vi "Acoustic Frequency Response Chirp.vi"(0 "TSM context":T1, 1 "dB SPL":dbl=94.0 format="%#_13g", 2 "Response Frequency (Hz)":dbl[](array[numeric])=[300.0, 18000.0], 5 "Start Freq (Hz)":dbl=20.0 format="%#_13g", 7 "Stop Freq (Hz)":dbl=20000.0 format="%#_13g", 9 "Samples":i32=128) -> (15 "error out":errorcluster)   [LabVIEW 2020]
doc: "VI performs an Acoustic Frequency Test with Calibrated Chirp waveform as input stimulus to microphone to obtain the equivalent Voltage Amplitude at given Frequencies."
uses:
  <vilib>/NI_TestStand_SemiconductorModule/NI_TestStand_Semiconductor_Module.lvlibp/PinMap/General/SemiconductorModuleContext.ctl
  e949006d-0b04-4f52-9731-e8b82caba12d.vi
  4e50633a-216a-4e31-9721-602c2020261f.vi
  c74fba9a-7462-4997-8ba2-8448d8120d66.vi
  f7f5d33f-d09a-4d82-ae73-b91c36f905d8.vi
  85eadde2-c8f2-4106-bb4c-7373345d24d2.vi
  28004d85-2d46-4c01-a9b5-50f3a10d13bf.vi
  e949006d-0b04-4f52-9731-e8b82caba12d.vi/1878dca8-edba-410e-aa20-92364f789876.vi
  4e50633a-216a-4e31-9721-602c2020261f.vi/75bb260e-55ca-447c-884a-a6f6cf63e709.vi
  <vilib>/measure/matone.llb/Extract Single Tone Information N Chan.vi
  <vilib>/NI_TestStand_SemiconductorModule/NI_TestStand_Semiconductor_Module.lvlibp/PinMap/General/Publish/PublishDataDoubleFunctionalTest.vi
  <vilib>/NI_TestStand_SemiconductorModule/NI_TestStand_Semiconductor_Module.lvlibp
  <vilib>/measure/NI_MAPro.lvlib
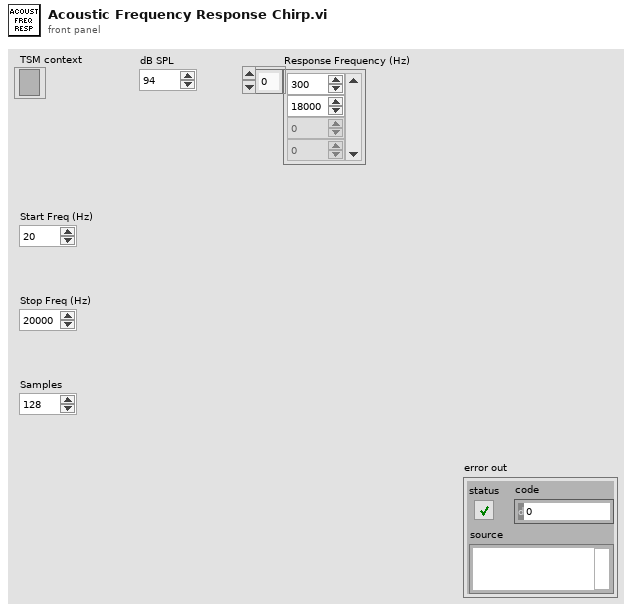
[diagram p1: front panel]
types:
  T1 = typedef "NI_TestStand_Semiconductor_Module.lvlibp/SemiconductorModuleContext.ctl" = refnum<k7>
  T2 = typedef "TSM DAQmx Multi-Task.ctl" = cluster{"Pin Query Context":refnum<class "MultiplePinMultipleSessionQueryContext.lvclass">, "SSC":T3[], "Site Numbers":i32[], "Pins":tag[]}
  T3 = typedef "SSC DAQmx.ctl" = cluster{"DAQmx Task ":refnum<k21>, "Channels":string, "Channel Lists":string}
  T4 = cluster{"approx freq. (optional)":dbl, "search (+/- % of Fsampl.)":dbl}
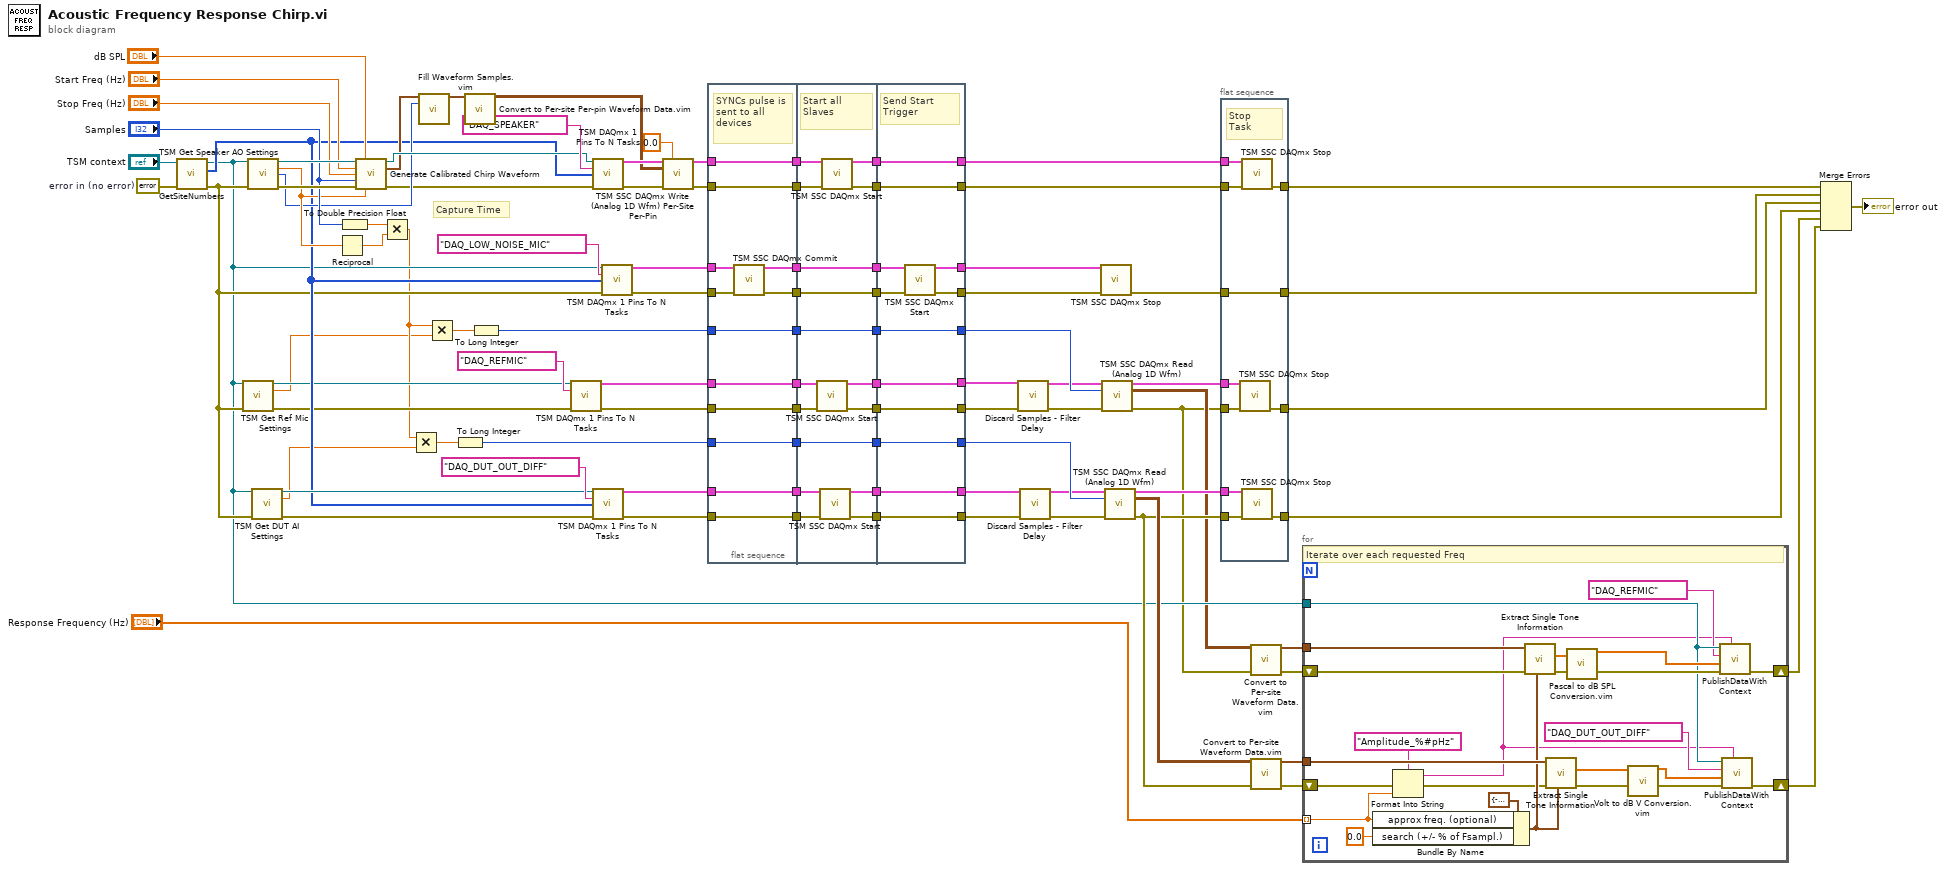
[diagram p0: block diagram]
diagram:
  w73 = errorcluster {"status"=FALSE, "code"=0, "source"=""}  # error in (no error)
  # "Capture Time"
  n1 = call <vilib>:"GetSiteNumbers.vi"("error in (no error)"=w73, "Semiconductor Module Context"="TSM context") -> ("error out"=w33:errorcluster, "Site Numbers"=w36:i32[], "Semiconductor Module Context Out"=w32:T1)  [unwired: 6 in, 1 out]
  n2 = call "TSM Get Ref Mic Settings.vi"("TSM context"=w32, "error in (no error)"=w33) -> ("TSM context Out"=w28:T1, "Sampling Rate (Hz)"=w25:dbl, "error out"=w30:errorcluster)  [unwired: 8 in, 3 out]
  n3 = call "TSM Get Speaker AO Settings.vi"("TSM context"=w32, "error in (no error)"=w33) -> ("TSM context Out"=w70:T1, "Sampling Rate (Hz)"=w64:dbl, "Samples per channel"=w38:i32, "error out"=w71:errorcluster)  [unwired: 9 in, 1 out]
  n4 = call "TSM Get DUT AI Settings.vi"("TSM context"=w32, "error in (no error)"=w33) -> ("TSM context Out"=w82:T1, "Sampling Rate (Hz)"=w35:dbl, "error out"=w81:errorcluster)  [unwired: 9 in, 2 out]
  n5 = Reciprocal(x=w64) -> (1/x=w78:dbl)
  n6 = To Double Precision Float(number="Samples") -> (double precision float=w77:dbl)
  n7 = call "Generate Calibrated Chirp Waveform.vi"("TSM context In"=w70, "dB SPL"="dB SPL", "Start Freq (Hz)"="Start Freq (Hz)", "Stop Freq (Hz)"="Stop Freq (Hz)", "Samples"="Samples", "error in (no error)"=w71, "Sampling Rate (Hz)"=w64) -> ("TSM context Out"=w69:T1, "Per Site Waveform"=w40:waveform(dbl)[], "error out"=w37:errorcluster)  [unwired: 6 in]
  n8 = Multiply(x=w77, y=w78) -> (x*y=w26:dbl)
  n9 = Multiply(x=w26, y=w35) -> (x*y=w34:dbl)
  n10 = call "Fill Waveform Samples.vim"("Waveform In"=w40, "Total Expected Samples"=w38) -> ("Waveform out"=w39:waveform(dbl)[])  [unwired: 13 in]
  n11 = Multiply(x=w26, y=w25) -> (x*y=w27:dbl)
  n12 = To Long Integer(number=w34) -> (32bit integer=w74:i32)
  n13 = call "Convert to Per-site Per-pin Waveform Data.vim"("Waveform In"=w39) -> ("Per Site Per Pin Waveform Out"=w41:waveform(dbl)[][])  [unwired: 14 in]
  n14 = To Long Integer(number=w27) -> (32bit integer=w22:i32)
  n15 = call "TSM DAQmx 1 Pins To N Tasks.vi"("TSM context"=w28, "Pins"=tag "DAQ_REFMIC", "error in"=w30) -> ("DAQ TSM Out"=w21:T2, "error out"=w29:errorcluster)  [unwired: 11 in]
  n16 = call "TSM DAQmx 1 Pins To N Tasks.vi"("TSM context"=w69, "Pins"=tag "DAQ_SPEAKER", "Site Numbers"=w36, "error in"=w37) -> ("DAQ TSM Out"=w83:T2, "error out"=w84:errorcluster)  [unwired: 10 in]
  n17 = call "TSM DAQmx 1 Pins To N Tasks.vi"("TSM context"=w82, "Pins"=tag "DAQ_DUT_OUT_DIFF", "Site Numbers"=w36, "error in"=w81) -> ("DAQ TSM Out"=w61:T2, "error out"=w80:errorcluster)  [unwired: 10 in]
  n18 = call "TSM DAQmx 1 Pins To N Tasks.vi"("TSM context"=w32, "Pins"=tag "DAQ_LOW_NOISE_MIC", "Site Numbers"=w36, "error in"=w33) -> ("DAQ TSM Out"=w62:T2, "error out"=w63:errorcluster)  [unwired: 10 in]
  n19 = call "TSM SSC DAQmx Write (Analog 1D Wfm) Per-Site Per-Pin.vi"("DAQ TSM in"=w83, "Idle Channel Value (0)"=0.0, "Per-Site Per-Pin Waveforms in"=w41, "error in"=w84) -> ("DAQ TSM Out"=w93:T2, "error out"=w79:errorcluster)  [unwired: 10 in]
  n20 = flat-sequence {
    tunnel: w74 -> [w105]
    tunnel: w93 -> [w106]
    tunnel: w79 -> [w107]
    tunnel: w61 -> [w108]
    tunnel: w80 -> [w109]
    tunnel: [w109] -> w60
    tunnel: [w108] -> w59
    tunnel: [w107] -> w58
    tunnel: [w106] -> w57
    tunnel: [w105] -> w56
    tunnel: w63 -> [w104]
    tunnel: w62 -> [w103]
    tunnel: [w102] -> w55
    tunnel: [w101] -> w54
    tunnel: w29 -> [w99]
    tunnel: [w100] -> w23
    tunnel: w22 -> [w100]
    tunnel: w21 -> [w98]
    tunnel: [w99] -> w20
    tunnel: [w98] -> w19
    tunnel: w60 -> [w120]
    tunnel: w59 -> [w119]
    tunnel: w58 -> [w125]
    tunnel: w57 -> [w123]
    tunnel: w56 -> [w121]
    tunnel: w55 -> [w116]
    tunnel: w54 -> [w115]
    tunnel: [w124] -> w53
    tunnel: [w122] -> w52
    tunnel: [w117] -> w51
    tunnel: [w118] -> w50
    tunnel: [w121] -> w49
    tunnel: [w116] -> w48
    tunnel: [w115] -> w47
    tunnel: [w114] -> w24
    tunnel: w23 -> [w114]
    tunnel: w20 -> [w113]
    tunnel: w19 -> [w112]
    tunnel: [w111] -> w18
    tunnel: [w110] -> w17
    tunnel: [w133] -> w75
    tunnel: [w134] -> w5
    tunnel: [w135] -> w92
    tunnel: [w136] -> w95
    tunnel: [w137] -> w94
    tunnel: w53 -> [w137]
    tunnel: w52 -> [w136]
    tunnel: w51 -> [w135]
    tunnel: w50 -> [w134]
    tunnel: w49 -> [w133]
    tunnel: w48 -> [w132]
    tunnel: w47 -> [w131]
    tunnel: [w130] -> w42
    tunnel: [w129] -> w44
    tunnel: [w128] -> w12
    tunnel: w24 -> [w128]
    tunnel: w18 -> [w127]
    tunnel: w17 -> [w126]
    tunnel: [w127] -> w16
    tunnel: [w126] -> w2
    frame #0 {
      # "SYNCs pulse is sent to all devices"
      n21 = call "TSM SSC DAQmx Commit.vi"("TSM DAQmx In"=w103, "error in (no error)"=w104) -> ("TSM DAQmx Out"=w101:T2, "error out"=w102:errorcluster)  [unwired: 12 in]
    }
    frame #1 {
      # "Start all Slaves"
      n22 = call "TSM SSC DAQmx Start.vi"("TSM DAQmx In"=w112, "error in (no error)"=w113) -> ("TSM DAQmx Out"=w110:T2, "error out"=w111:errorcluster)  [unwired: 12 in]
      n23 = call "TSM SSC DAQmx Start.vi"("TSM DAQmx In"=w119, "error in (no error)"=w120) -> ("TSM DAQmx Out"=w118:T2, "error out"=w117:errorcluster)  [unwired: 12 in]
      n24 = call "TSM SSC DAQmx Start.vi"("TSM DAQmx In"=w123, "error in (no error)"=w125) -> ("TSM DAQmx Out"=w122:T2, "error out"=w124:errorcluster)  [unwired: 12 in]
    }
    frame #2 {
      # "Send Start Trigger"
      n25 = call "TSM SSC DAQmx Start.vi"("TSM DAQmx In"=w131, "error in (no error)"=w132) -> ("TSM DAQmx Out"=w130:T2, "error out"=w129:errorcluster)  [unwired: 12 in]
    }
  }
  n26 = call "Discard Samples - Filter Delay.vi"("DAQ TSM in"=w2, "error in"=w16) -> ("DAQ TSM Out"=w1:T2, "error out"=w3:errorcluster)  [unwired: 12 in]
  n27 = call "Discard Samples - Filter Delay.vi"("DAQ TSM in"=w5, "error in"=w92) -> ("DAQ TSM Out"=w4:T2, "error out"=w6:errorcluster)  [unwired: 12 in]
  n28 = call "TSM SSC DAQmx Stop.vi"("TSM DAQmx In"=w42, "error in (no error)"=w44) -> ("error out"=w43:errorcluster)  [unwired: 12 in, 1 out]
  n29 = call "TSM SSC DAQmx Read (Analog 1D Wfm).vi"("DAQ TSM in"=w1, "Samples to read"=w12, "error in"=w3) -> ("DAQ TSM Out"=w13:T2, "Per-Site Per-Pin Waveforms Out"=w11:waveform(dbl)[][], "error out"=w9:errorcluster)  [unwired: 10 in]
  n30 = call "TSM SSC DAQmx Read (Analog 1D Wfm).vi"("DAQ TSM in"=w4, "Samples to read"=w75, "error in"=w6) -> ("DAQ TSM Out"=w91:T2, "Per-Site Per-Pin Waveforms Out"=w90:waveform(dbl)[][], "error out"=w86:errorcluster)  [unwired: 10 in]
  n31 = flat-sequence {
    tunnel: w95 -> [w147]
    tunnel: w94 -> [w146]
    tunnel: w91 -> [w145]
    tunnel: w86 -> [w144]
    tunnel: [w143] -> w15
    tunnel: [w142] -> w89
    tunnel: [w141] -> w46
    tunnel: w43 -> [w141]
    tunnel: w9 -> [w140]
    tunnel: [w139] -> w14
    tunnel: w13 -> [w138]
    frame #0 {
      # "Stop \nTask"
      n32 = call "TSM SSC DAQmx Stop.vi"("TSM DAQmx In"=w138, "error in (no error)"=w140) -> ("error out"=w139:errorcluster)  [unwired: 12 in, 1 out]
      n33 = call "TSM SSC DAQmx Stop.vi"("TSM DAQmx In"=w147, "error in (no error)"=w146) -> ("error out"=w142:errorcluster)  [unwired: 12 in, 1 out]
      n34 = call "TSM SSC DAQmx Stop.vi"("TSM DAQmx In"=w145, "error in (no error)"=w144) -> ("error out"=w143:errorcluster)  [unwired: 12 in, 1 out]
    }
  }
  n35 = call "Convert to Per-site Waveform Data.vim"("Per-Site Per-Pin Waveform In"=w11) -> ("Per-Site Waveform Out"=w10:waveform(dbl)[])  [unwired: 14 in]
  n36 = call "Convert to Per-site Waveform Data.vim"("Per-Site Per-Pin Waveform In"=w90) -> ("Per-Site Waveform Out"=w87:waveform(dbl)[])  [unwired: 14 in]
  n37 = for {
    tunnel: w87 -> [w169]
    shift-right: [w165] -> w8
    shift-left: w86 -> [w156]
    tunnel: "Response Frequency (Hz)" -> [w163] mode=indexing
    tunnel: w32 -> [w151]
    tunnel: w10 -> [w161]
    shift-right: [w157] -> w7
    shift-left: w9 -> [w158]
    # "Iterate over each requested Freq"
    n38 = Bundle By Name(cluster=T4 {"approx freq. (optional)"=-1.0, "search (+/- % of Fsampl.)"=5.0} ("advanced search"), "approx freq. (optional)"=w163, "search (+/- % of Fsampl.)"=0.0) -> (w162:T4)
    n39 = Format Into String(format string="Amplitude_%#pHz", error in=w156, w163) -> (resulting string=w148:string, error out=w160:errorcluster)  [unwired: 1 in]
    n40 = call-poly <vilib>:"Extract Single Tone Information.vi"("advanced search"=w162, "error in (no error)"=w158, "time signals in"=w161) -> ("error out"=w159:errorcluster, "detected amplitudes"=w155:dbl[])  [unwired: 3 in, 4 out]
    n41 = call-poly <vilib>:"Extract Single Tone Information.vi"("advanced search"=w162, "error in (no error)"=w160, "time signals in"=w169) -> ("error out"=w166:errorcluster, "detected amplitudes"=w153:dbl[])  [unwired: 3 in, 4 out]
    n42 = call "Pascal to dB SPL Conversion.vim"("Pascals"=w155) -> ("dbSPL"=w154:dbl[])  [unwired: 14 in]
    n43 = call "Volt to dB V Conversion.vim"("Voltage"=w153) -> ("dB V"=w152:dbl[])  [unwired: 14 in]
    n44 = call-poly <vilib>:"PublishDataWithContext.vi"("Published Data Id"=w148, "error in (no error)"=w159, "Data In"=w154, "Pin"=tag "DAQ_REFMIC" ("Pins"), "Semiconductor Module Context"=w151) -> ("error out"=w157:errorcluster)  [unwired: 5 in, 1 out]
    n45 = call-poly <vilib>:"PublishDataWithContext.vi"("Published Data Id"=w148, "error in (no error)"=w166, "Data In"=w152, "Pin"=tag "DAQ_DUT_OUT_DIFF" ("Pins"), "Semiconductor Module Context"=w151) -> ("error out"=w165:errorcluster)  [unwired: 5 in, 1 out]
  }
  n46 = Merge Errors(w89, w46, w14, w15, w7, w8) -> (→"error out":errorcluster)
